vi "Database Example.vi"() -> ()   [LabVIEW 2019]
doc: "Shows an example using a SQLite Database as the output sink for log events."
uses:
  Log/Event Level.ctl
  Log/Log.lvclass/Log.ctl
  Layouts/JSONLayout/JSONLayout.lvclass
  C:/Development/Open Source/tsc-event-logger/Layouts/Layout.lvclass
  cd0cdadd-5bba-4876-b4a7-6d6dc25bebc9.vi
  0255d82c-ae35-4f1c-bf70-cf29c14a7855.vi
  d915b4c3-683c-4e5b-a72c-46a47fdfc3fe.vi
  Log/Read Sinks.vi
  Log Sinks/SQLite Database/SQLite Database.lvclass
  C:/Development/Open Source/tsc-event-logger/Log Sinks/Log Sinks.lvclass
  Log Sinks/Sink-Console/Sink-Console.lvclass
  Log Sinks/Send Log Packet.vi
  Log/Log.lvclass
  TSC Event Logger.lvlib
panel:
  in  "Record Event with multiple arg":bool
  in  "Record Event with arg":bool
  in  "Argument List":string[](array[string])
  in  "Single Argument":string
  in  "Add JSON Console":bool
  out "Second Console":string
  out "String":string
  in  "Level":T1=enum."INFO"
  in  "Record Event":bool
  in  "Event Data":string="test"
  out "Error Out":errorcluster
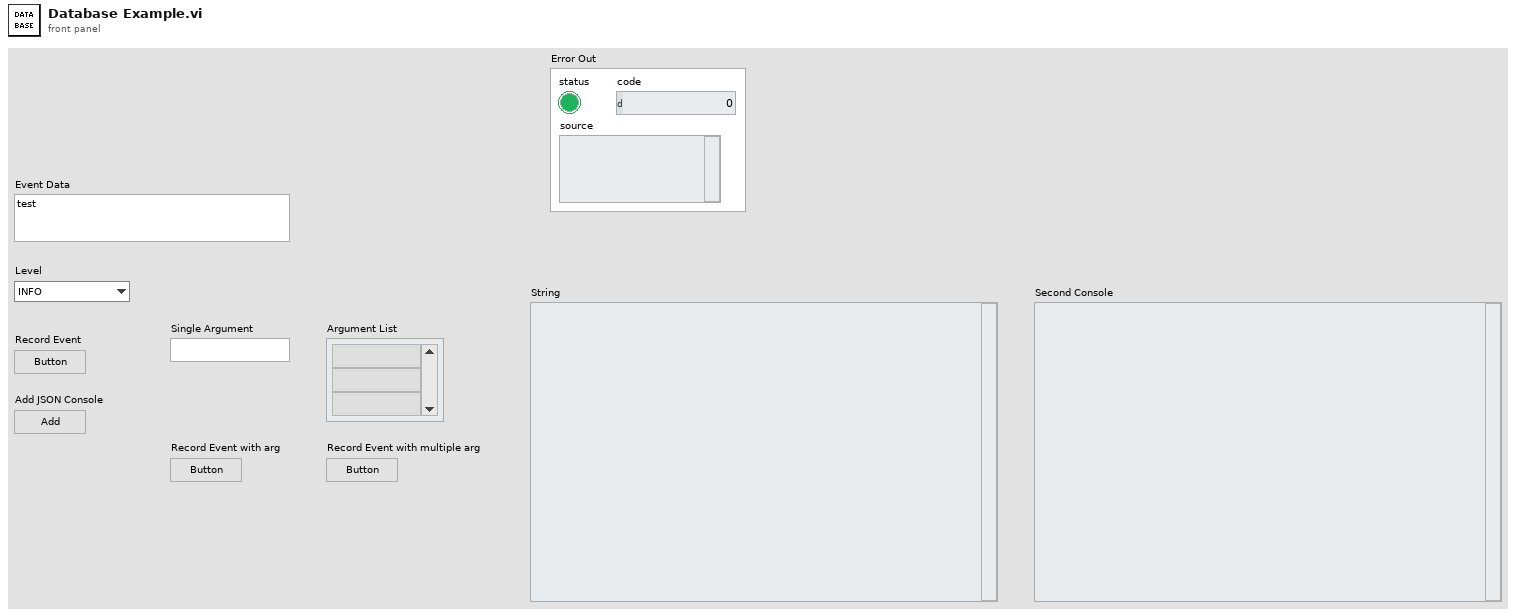
[diagram p1: front panel]
types:
  T1 = typedef "TSC Event Logger.lvlib/Event Level.ctl" = enum16{"OFF", "TRACE", "DEBUG", "INFO", "WARN", "ERROR", "FATAL"}
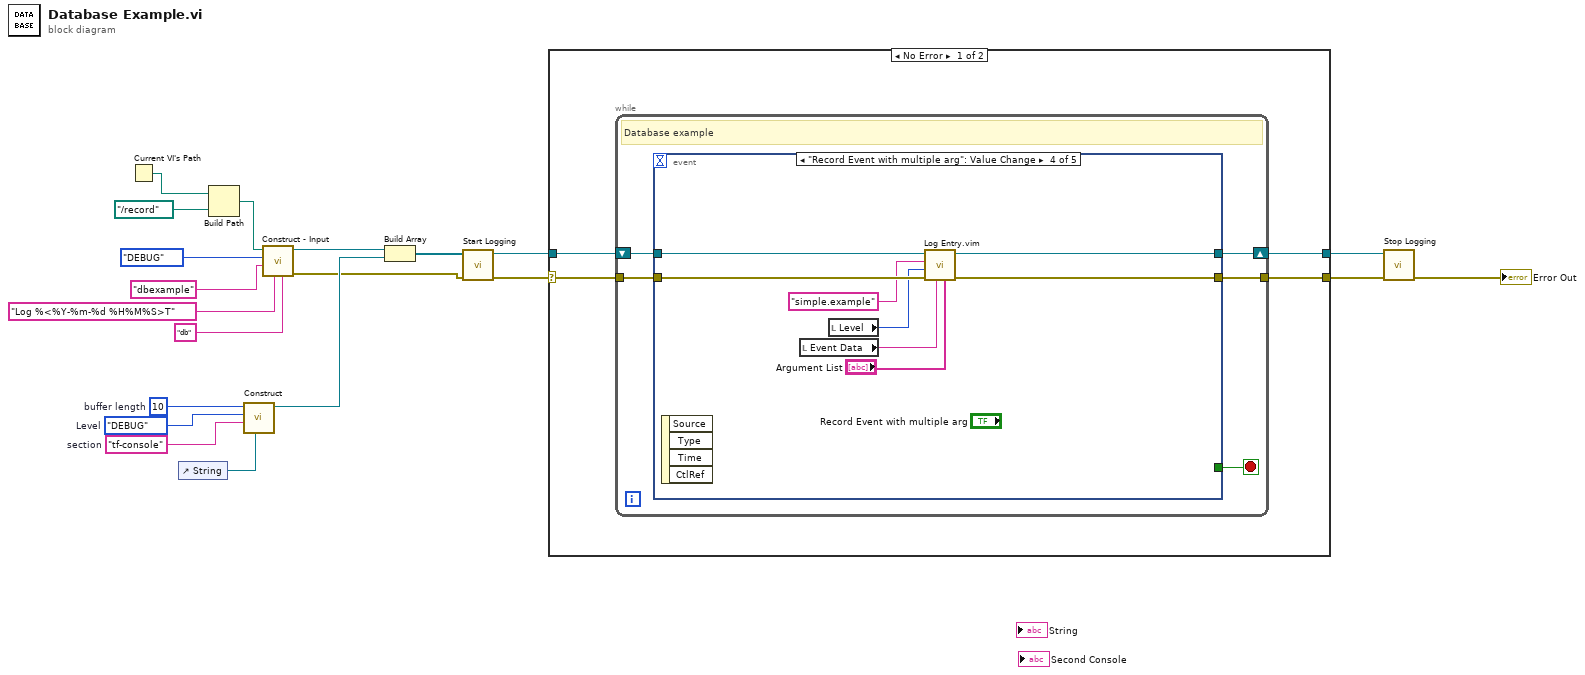
[diagram p0: block diagram]
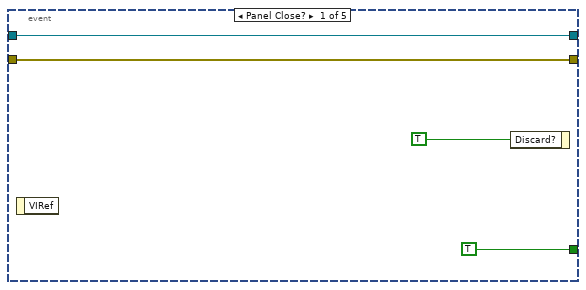
[diagram p2: hidden frame]
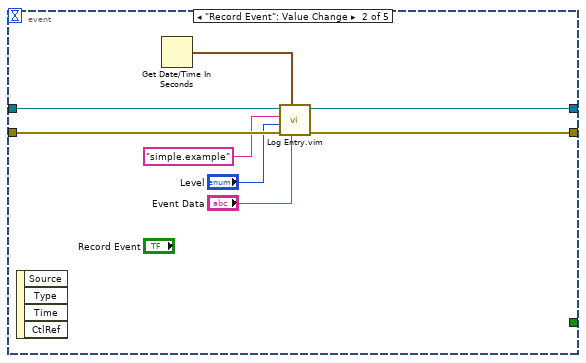
[diagram p3: hidden frame]
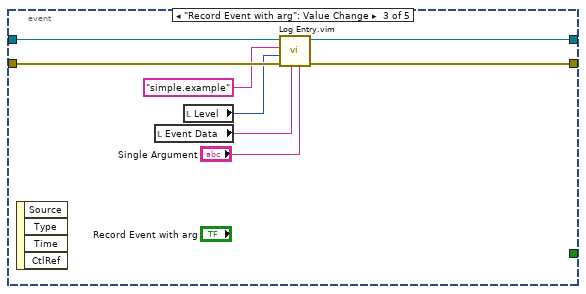
[diagram p4: hidden frame]
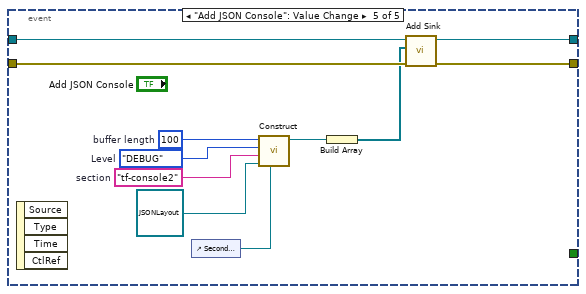
[diagram p5: hidden frame]
diagram:
  w8 = 10  # buffer length
  w9 = Event_Level."DEBUG"  # Level
  w10 = "tf-console"  # section
  n1 = Current VI's Path() -> (path=w1:path)
  n2 = control-ref of="String"() -> (w11:refnum<vi>)
  n3 = Build Path(base path=w1, name or relative path=path "../record") -> (appended path=w13:path)
  n4 = call-poly "Construct.vi"("Console Ref"=w11, "Name"=w10, "Level"=w9, "buffer length"=w8) -> ("Sink-Console"=w12:refnum<class "Sink-Console.lvclass">)  [unwired: 6 in, 1 out]
  n5 = call "Construct - Input.vi"("extension"="db", "file name format"="Log %<%Y-%m-%d %H%M%S>T", "Name"="dbexample" ("section"), "Level"=Event_Level."DEBUG", "log location"=w13) -> ("error out"=w3:errorcluster, "SQLite Database out"=w16:refnum<class "SQLite Database.lvclass">)  [unwired: 5 in]
  n6 = Build Array(w16, w12) -> (w15:refnum<class "Log Sinks.lvclass">[])
  n7 = call "Start Logging.vi"("Error In"=w3, "Sinks"=w15) -> ("Error Out"=w2:errorcluster, "Logger"=w17:refnum<class "Log.lvclass">)  [unwired: 8 in]
  n8 = case shown="No Error" w2 {
    selector: w2 -> [w21 w70]
    tunnel: [w24 w69] -> w19
    tunnel: [w23 w70] -> w18
    tunnel: w17 -> [w22 w69]
    frame No Error {
      n9 = while {
        tunnel: w21 -> [w28]
        shift-right: [w26] -> w24
        shift-left: w22 -> [w27]
        tunnel: [w25] -> w23
        stop <- w29 stop-if-true
        # "Database example"
        n10 = event shown="[3] \"Record Event with multiple arg\": Value Change" {
          selector: _ -> [_ _ _ _ _]
          dyn-events: _ -> [_ _ _ _ _]
          timeout: _ -> [_ _ _ _ _]
          tunnel: [TRUE _ _ _ _] -> w29
          tunnel: w28 -> [w30 w39 w47 w55 w68]
          tunnel: w27 -> [w31 w41 w49 w57 w66]
          tunnel: [w31 w40 w48 w56 w65] -> w26
          tunnel: [w30 w38 w46 w54 w67] -> w25
          event Panel Close? {
            n11 = event-data() -> ()  [unwired: 1 in, 1 out]
            n12 = event-data("Discard?"=TRUE) -> ()  [unwired: 1 in, 1 out]
          }
          event "Record Event": Value Change {
            n13 = event-data() -> ()  [unwired: 1 in, 4 out]
            n14 = Get Date/Time In Seconds() -> (seconds since 1Jan1904=w36:timestamp)
            n15 = call "Log Entry.vim"("Message"="Event Data", "Time"=w36, "error in (no error)"=w39, "Level"="Level", "Logger"="simple.example", "Log in"=w41) -> ("error out"=w38:errorcluster, "Log out"=w40:refnum<class "Log.lvclass">)  [unwired: 4 in]
          }
          event "Record Event with arg": Value Change {
            n16 = event-data() -> ()  [unwired: 1 in, 4 out]
            n17 = local read "Event Data"() -> (w43:string)
            n18 = local read "Level"() -> (w44:T1)
            n19 = call "Log Entry.vim"("Arguments"="Single Argument", "Message"=w43, "error in (no error)"=w47, "Level"=w44, "Logger"="simple.example", "Log in"=w49) -> ("error out"=w46:errorcluster, "Log out"=w48:refnum<class "Log.lvclass">)  [unwired: 4 in]
          }
          event "Record Event with multiple arg": Value Change {
            n20 = event-data() -> ()  [unwired: 1 in, 4 out]
            n21 = local read "Event Data"() -> (w51:string)
            n22 = local read "Level"() -> (w52:T1)
            n23 = call "Log Entry.vim"("Arguments"="Argument List", "Message"=w51, "error in (no error)"=w55, "Level"=w52, "Logger"="simple.example", "Log in"=w57) -> ("error out"=w54:errorcluster, "Log out"=w56:refnum<class "Log.lvclass">)  [unwired: 4 in]
          }
          event "Add JSON Console": Value Change {
            w64 = 100  # buffer length
            w63 = Event_Level."DEBUG"  # Level
            w62 = "tf-console2"  # section
            n24 = event-data() -> ()  [unwired: 1 in, 4 out]
            n25 = control-ref of="Second Console"() -> (w61:refnum<vi>)
            n26 = call-poly "Construct.vi"("Console Ref"=w61, "Layout Type"=refnum<class "JSONLayout.lvclass"> refnum ("TSC Event Logger.lvlib:JSONLayout.lvclass"), "Name"=w62, "Level"=w63, "buffer length"=w64) -> ("Sink-Console"=w60:refnum<class "Sink-Console.lvclass">)  [unwired: 5 in, 1 out]
            n27 = Build Array(w60) -> (w59:refnum<class "Sink-Console.lvclass">[])
            n28 = call "Add Sink.vi"("Error In"=w68, "Sinks"=w59, "Logger in"=w66) -> ("Error Out"=w67:errorcluster, "Logger"=w65:refnum<class "Log.lvclass">)  [unwired: 7 in]
          }
        }
      }
    }
    frame Error {
    }
  }
  n29 = call "Stop Logging.vi"("Error In"=w18, "Logger"=w19) -> ("Error Out"=→"Error Out":errorcluster)  [unwired: 8 in, 1 out]
